vi "Enclose Selection And Move.vi"   [LabVIEW 2019]
doc: "Demonstrates the Enclose Selection 2 method in VI Scripting to enclose a selection of block diagram objects within a structure, then move that structure to a different VI.\n\nThe Enclose Selection 2 method can make it easy to move multiple objects. Unlike the Move Selection method, wires between the selected objects don't have to be individually selected in order to maintain connections between nodes."
uses:
  <vilib>/Utility/miscctls.llb/LVPositionTypeDef.ctl
  <vilib>/Utility/traverseref.llb/TRef TravTarget.ctl
  <vilib>/Utility/traverseref.llb/VI Scripting - Traverse.lvlib
panel:
  # "Overview: Demonstrates the Enclose Selection 2 method in VI Scripting to programmatically create a structure around the selected part of the block diagram.\nInstructions:\n1. Open the block diagrams of Test - Moving Objects Source.vi and Test - Moving Objects Target.vi.\n2. Select at least one object on the diagram of the Source VI.\n3. Run this VI. The item(s) you selected will be wrapped in a Sequence structure, and moved to the Target VI.\n\nNote: When moving an object from one VI to another, the operation results in a copy, since the original object is preserved. When moving an object to a different location in the same VI, it will not be a copy operation unless the Duplicate? parameter of the Move method is set to TRUE."
types:
  T1 = typedef "TRef TravTarget.ctl" = enum16{"FP", "BD", "Other"}
  T2 = typedef "LVPositionTypeDef.ctl" = cluster{"Left":i32, "Top":i32}
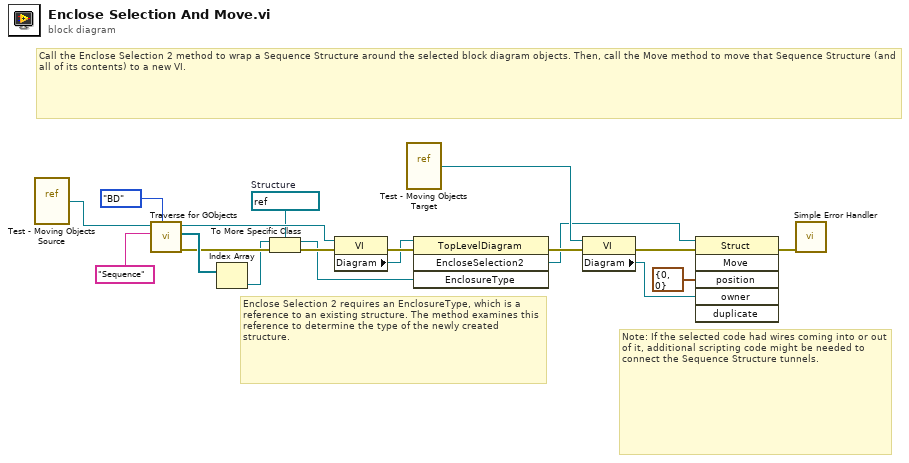
[diagram p0: block diagram]
diagram:
  w3 = refnum<vi> refnum  # Structure
  # "Call the Enclose Selection 2 method to wrap a Sequence Structure around the selected block diagram objects. Then, call the Move method to move that Sequence Structure (and all of its contents) to a new VI."
  # "Enclose Selection 2 requires an EnclosureType, which is a reference to an existing structure. The method examines this reference to determine the type of the newly created structure."
  # "Note: If the selected code had wires coming into or out of it, additional scripting code might be needed to connect the Sequence Structure tunnels."
  n1 = vi-ref "Test - Moving Objects Source.vi"() -> (w13:refnum<vi>)
  n2 = call <vilib>:"Traverse for GObjects.vi"("Traverse Target"=TRef_TravTarget."BD", "Class Name"="Sequence", "VI Refnum"=w13) -> ("error out"=w7:errorcluster, "References"=w8:refnum<vi>[], "dup VI Refnum"=w9:refnum<vi>)  [unwired: 5 in, 1 out]
  n3 = Index Array(array=w8) -> (element=w4:refnum<vi>)  [unwired: 1 in]
  n4 = To More Specific Class(target class=w3, reference=w4, error in=w7) -> (specific class reference=w5:refnum<vi>, error out=w6:errorcluster)
  n5 = property class="VI"(reference=w9, error in=w6) -> (error out=w12:errorcluster, "Diagram"=w2:refnum<vi>)  [unwired: 1 out]
  n6 = vi-ref "Test - Moving Objects Target.vi"() -> (w19:refnum<vi>)
  n7 = invoke class="TopLevelDiagram" method="EncloseSelection2"(reference=w2, error in=w12, "EnclosureType"=w5) -> (error out=w16:errorcluster, "EncloseSelection2"=w14:refnum<vi>)  [unwired: 1 in, 2 out]
  n8 = property class="VI"(reference=w19, error in=w16) -> (error out=w15:errorcluster, "Diagram"=w17:refnum<vi>)  [unwired: 1 out]
  n9 = invoke class="Struct" method="Move"(reference=w14, error in=w15, "position"=T2 {"Left"=0, "Top"=0}, "owner"=w17) -> (error out=w1:errorcluster)  [unwired: 2 in, 5 out]
  n10 = call <vilib>:"Simple Error Handler.vi"("error in (no error)"=w1) -> ()  [unwired: 4 in, 5 out]
